vi "LIA Basic SineCosine FPGA.vi"() -> ()   [LabVIEW 2017]
uses:
  <instrlib>/_niInstr/Streaming/v1/Common/Stream State.ctl
  <vilib>/Platform/TimedLoop/XDataNode/timing_clust.ctl
  <vilib>/Platform/TimedLoop/XDataNode/nitl_modes.ctl
  <vilib>/Platform/TimedLoop/XDataNode/wakeup.ctl
  <vilib>/rvi/FXPMathLib/FxpSinAndCos/subVIs/nifxpmath_SinAndCos_SimConfig.ctl
  <vilib>/rvi/Emulation/niFpgaSctlEmulationGetInTimedLoop.vi
  <vilib>/rvi/Emulation/niFpgaEmulationReportErrorSimple.vi
  <vilib>/rvi/Emulation/niFpgaGetClockAttributes.vi
  <vilib>/rvi/Emulation/niFpgaCriticalErrorInLSC.vi
  <vilib>/rvi/FXPMathLib/FxpSinAndCos/simVIs/DllFxpSinAndCosTemp_sub.vi
  <instrlib>/_niInstr/Basic Elements/v1/FPGA/Private/Count Up U64.vi
  <vilib>/rvi/interface/RandomDataEmulation/niFpgaRandomDataHandleErrors.vi
  <vilib>/Platform/TimedLoop/XDataNode/XDataNode.xnode
  <vilib>/rvi/FXPMathLib/FxpAdd/XNode/nifxpmath_Add.xnode
  <vilib>/rvi/FXPMathLib/FxpSinAndCos/XNode/nifxpmath_SinAndCos.xnode
  <vilib>/rvi/FXPMathLib/FxpMul/XNode/nifxpmath_Multiplier.xnode
  <vilib>/rvi/FXPMathLib/FxpSub/XNode/nifxpmath_Sub.xnode
  <vilib>/rvi/DataTransferAndStorage/Container/XNode/niFpgaContainer.xnode
  <vilib>/rvi/interface/RandomDataEmulation/nirviRandomDataFpgaReadWriteTemplate.vi
  <vilib>/Platform/TimedLoop/XDataNode/XDNodeRunTimeDep.lvlib
  <instrlib>/_niInstr/Streaming/v1/FPGA/niInstr Streaming v1 FPGA.lvlib
  <instrlib>/_niInstr/Basic Elements/v1/FPGA/niInstr Basic Elements v1 FPGA.lvlib
  <vilib>/rvi/FXPMathLib/sim/FxpSim.dll
  <instrlib>/_niInstr/Streaming/v1/Common/niInstr Streaming v1 Common.lvlib
panel:
  in  "fs?":bool
  out "SineCosine rdi count":u64
  in  "clear rdi counters (T) 0":bool=TRUE
  out "FIFO rdi count":u64
  in  "stream.num samples 0":u64
  in  "stream.request state 0":T1
  out "stream.state 0":T1
  out "stream.samples transferred 0":u64
  out "stream.metadata 0":u64
  in  "strem.force error 0":bool caption="force error (false)"
  in  "phase delta (pi rad)":fxp<+/-,20,1>
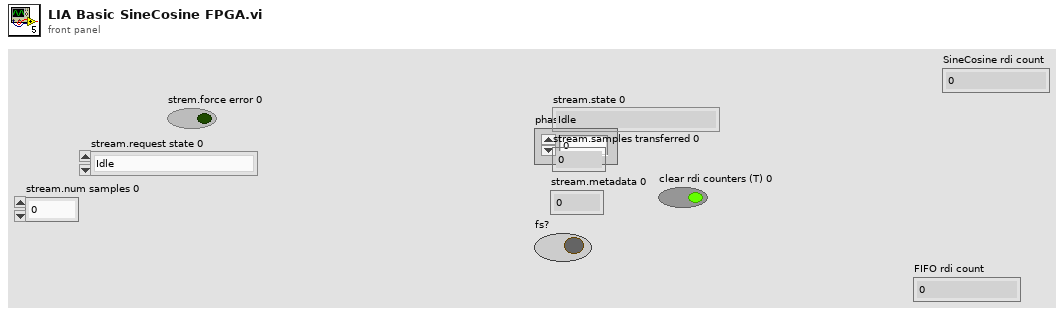
[diagram p1: front panel]
types:
  T1 = typedef "niInstr Streaming v1 Common.lvlib/Stream State.ctl" = enum8{"Idle", "Finite Transfer", "Continuous", "Done", "Error", "Not Ready", "Cancel"}
  T2 = typedef "XDNodeRunTimeDep.lvlib/timing_clust.ctl" = cluster{"Expected End [f-1]":u64, "Actual End [f-1]":u64, "Finished Late? [f-1]":bool, "Expected End [i-1]":u64, "Actual End [i-1]":u64, "Finished Late? [i-1]":bool, "Expected Start [i]":u64, "Actual Start [i]":u64, "Expected Start [f]":u64, "Actual Start [f]":u64, "Source Name":string, "Structure Name":string, "Period":i64, "Deadline":i64, "Offset":i64, "Start":i64, "Priority":i32, "Timeout":i32, "Mode":T3, "Wakeup Reason":T4, "Error":errorcluster, "Source Type":string, "Secondary Source Type":string, "Global End Time":u64, "Global Start Time":u64, "Frame Duration":u64, "Iteration Duration":u64, "Assigned CPU":i32, "I/O Scan Engine Mode":u32}
  T3 = typedef "XDNodeRunTimeDep.lvlib/nitl_modes.ctl" = enum32{"No Change", "Process missed periods, maintain original phase", "Discard missed periods, maintain original phase", "Process missed periods, ignore original phase", "Discard missed periods, ignore original phase"}
  T4 = typedef "XDNodeRunTimeDep.lvlib/wakeup.ctl" = enum32{"Normal", "Aborted", "Asynchronous wakeup", "Timing source error", "Timed loop error", "Timeout"}
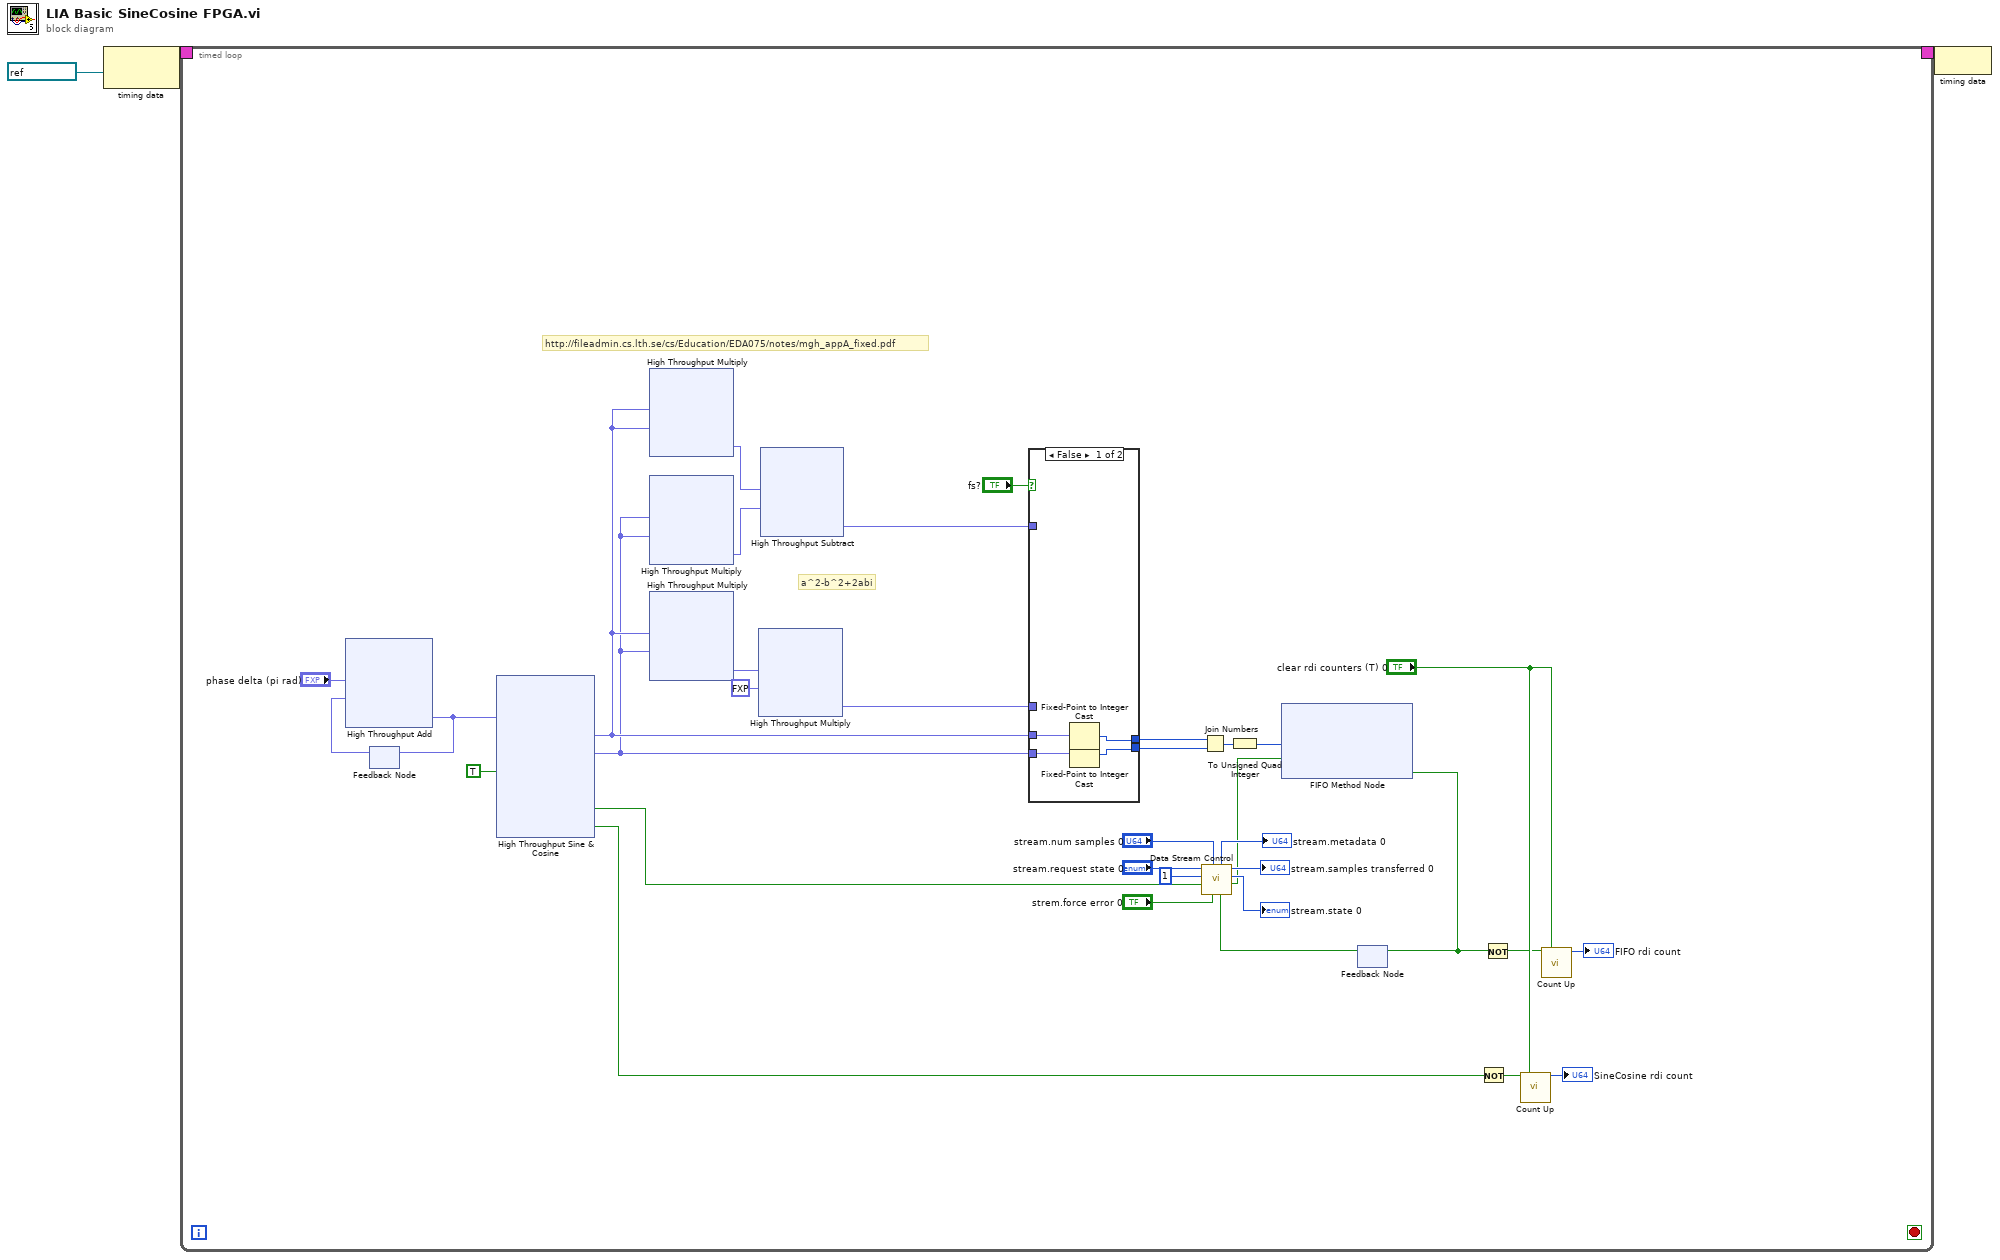
[diagram p0: block diagram]
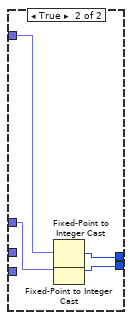
[diagram p2: hidden frame]
diagram:
  n1 = node-c288(refnum<k21> "100MHz" ("Source Name")) -> (w3:T2)
  n2 = timed-loop {
    timing: w3 -> [_]
    timing-out: [_] -> w2
    stop <- _ stop-if-true
    # "a^2-b^2+2abi"
    # "http://fileadmin.cs.lth.se/cs/Education/EDA075/notes/mgh_appA_fixed.pdf"
    n3 = feedback #1() -> (w36:fxp<+/-,22,2>)  [unwired: 1 in]
    n4 = xnode ("High Throughput Add")("x"="phase delta (pi rad)", "y"=w36) -> ("x+y"=w35:fxp<+/-,22,2>)
    n5 = feedback-in #1(w35) -> ()
    n6 = xnode "High Throughput Sine & Cosine"("x (pi)"=w35, "input valid"=TRUE) -> ("sin(x)"=w11:fxp<+/-,21,2>, "cos(x)"=w10:fxp<+/-,21,2>, "output valid"=w24:bool, "ready for input"=w19:bool)  [unwired: 1 in]
    n7 = xnode ("High Throughput Multiply")("x"=w11, "y"=w11) -> ("x*y"=w9:fxp<+/-,20,2>)
    n8 = xnode ("High Throughput Multiply")("x"=w10, "y"=w10) -> ("x*y"=w8:fxp<+/-,20,2>)
    n9 = xnode ("High Throughput Multiply")("x"=w11, "y"=w10) -> ("x*y"=w14:fxp<+/-,20,2>)
    n10 = xnode ("High Throughput Multiply")("x"=w14, "y"=fxp<+,2,2> 2.0) -> ("x*y"=w12:fxp<+/-,22,4>)
    n11 = xnode ("High Throughput Subtract")("x"=w9, "y"=w8) -> ("x-y"=w7:fxp<+/-,21,3>)
    n12 = case shown="False" "fs?" {
      tunnel: w7 -> [_ w42]
      tunnel: w11 -> [w41 _]
      tunnel: w10 -> [w40 _]
      tunnel: [w39 w45] -> w16
      tunnel: [w38 w44] -> w15
      tunnel: w12 -> [_ w43]
      frame False {
        n13 = Fixed-Point to Integer Cast(1:w41) -> (0:w39:i32)
        n14 = Fixed-Point to Integer Cast(1:w40) -> (0:w38:i32)
      }
      frame True {
        n15 = Fixed-Point to Integer Cast(1:w42) -> (0:w45:i32)
        n16 = Fixed-Point to Integer Cast(1:w43) -> (0:w44:i32)
      }
    }
    n17 = Join Numbers(hi=w16, lo=w15) -> ((hi.lo)=w34:u64)
    n18 = To Unsigned Quad Integer(1:w34) -> (0:w33:u64)
    n19 = feedback #2() -> (w23:bool)  [unwired: 1 in]
    n20 = call <instrlib>:"Data Stream Control.vi"("ready for input?"=w23, "force error"="strem.force error 0", "stream.num samples 0"="stream.num samples 0", "data valid"=w24, "element count"=u16 1, "stream.request state 0"="stream.request state 0") -> ("send data"=w25:bool, "stream.state 0"=→"stream.state 0":T1, "stream.samples transferred 0"=→"stream.samples transferred 0":u64, "stream.metadata 0"=→"stream.metadata 0":u64)  [unwired: 1 in, 1 out]
    n21 = xnode ("FIFO Method Node")("Element"=w33, "Input Valid"=w25) -> ("Ready for Input"=w21:bool)  [unwired: 1 in, 1 out]
    n22 = feedback-in #2(w21) -> ()
    n23 = Not(x=w19) -> (.not. x?=w4:bool)
    n24 = Not(x=w21) -> (.not. x?=w5:bool)
    n25 = call-poly <instrlib>:"Count Up.vi"("increment"=w4, "reset"="clear rdi counters (T) 0") -> ("count out"=→"SineCosine rdi count":u64)  [unwired: 13 in]
    n26 = call-poly <instrlib>:"Count Up.vi"("increment"=w5, "reset"="clear rdi counters (T) 0") -> ("count out"=→"FIFO rdi count":u64)  [unwired: 13 in]
  }
  n27 = node-c288(w2) -> ()
